vi "Status_Error_Message.vi"(1 "Message number":i32 min=0 step=1) -> (0 "Status/Error string":string)   [LabVIEW 2012]
uses:
  Globals/Status_Error_Messages.vi
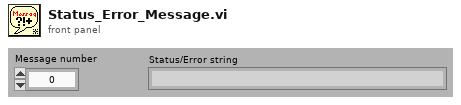
[diagram p1: front panel]
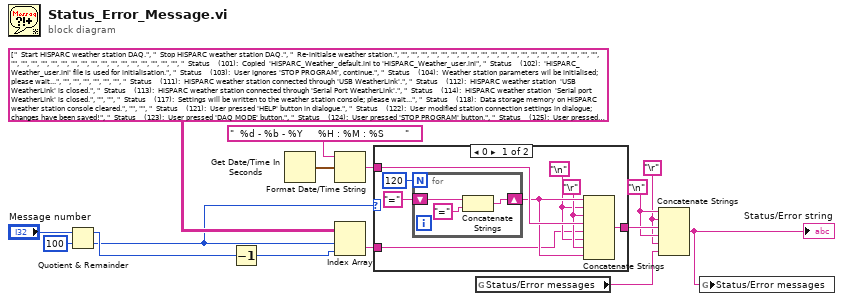
[diagram p0: block diagram]
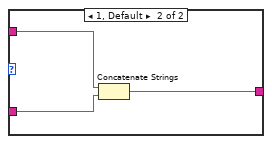
[diagram p2: hidden frame]
diagram:
  w11 = "\n"
  w10 = "\r"
  n1 = Quotient & Remainder(x="Message number", y=100) -> (x-y*floor(x/y)=w5:i32, floor(x/y)=w1:i32)
  n2 = Decrement(x=w5) -> (x-1=w2:i32)
  n3 = Get Date/Time In Seconds() -> (seconds since 1Jan1904=w15:timestamp)
  n4 = Format Date/Time String(time format string (%c)="  %d - %b - %Y     %H : %M : %S       ", seconds (now)=w15) -> (date/time string=w13:string)  [unwired: 1 in]
  n5 = Index Array(array=string[][] [["  Start HiSPARC weather station DAQ.", "  Stop HiSPARC weather station DAQ.", "  Re-initialse weather station.", "", "", "", "", "", "", "", "", "", "", "", "", "", "", "", "", "", "", "", "", "", "", "", "", "", "", "", "", "", "", "", "", "", "", "", "", ""], ["  Status    (101):  Copied  'HiSPARC_Weather_default.ini to 'HiSPARC_Weather_user.ini", "  Status    (102):  'HiSPARC_Weather_user.ini' file is used for initialisation.", "  Status    (103):  User ignores 'STOP PROGRAM', continue.", "  Status    (104):  Weather station parameters wil be initialised; please wait...", "", "", "", "", "", "", "  Status    (111):  HiSPARC weather station connected through 'USB WeatherLink'.", "  Status    (112):  HiSPARC weather station  'USB WeatherLink' is closed.", "  Status    (113):  HiSPARC weather station connected through 'Serial Port WeatherLink'.", "  Status    (114):  HiSPARC weather station  'Serial port WeatherLink' is closed.", "", "", "  Status    (117):  Settings will be written to the weather station console; please wait...", "  Status    (118):  Data storage memory on HiSPARC weather station console cleared.", "", "", "  Status    (121):  User pressed 'HELP' button in dialogue.", "  Status    (122):  User modified station connection settings in dialogue; changes have been saved!", "  Status    (123):  User pressed 'DAQ MODE' button.", "  Status    (124):  User pressed 'STOP PROGRAM' button.", "  Status    (125):  User pressed 'SAVE SETTINGS' button.", "  Status    (126):  User pressed 'SAVE CALIBRATION' button; please wait until settings have been uploaded...", "  Status    (127):  User skips weather station calibration, continue.", "  Status    (128):  User pressed 'RESET' button but skips reset.", "  Status    (129):  User pressed 'HELP' button.", "  Status    (130):  User pressed 'STOP DAQ' button.", "  Status    (131):  Weather station console successfully initialised.", "", "", "", "", "  Status    (136):  Calibration: latitude and longitude have not been modified.", "  Status    (137):  Calibration: temperature and/or humidity settings have not been modified.", "", "  Status    (139):  Calibration: wind direction has not been modified.", "  Status    (140):  Calibration: barometer settings have not been modified."], ["  Warning (201):  No GPS time correction in HiSPARC.ini (correction = 0)!", "", "", "", "", "", "", "", "", "", "  Warning (211):  Cannot open HiSPARC weather station connection through 'USB WeatherLink'!", "  Warning (212):  Cannot close HiSPARC weather station connection through 'USB WeatherLink'", "  Warning (213):  Cannot open HiSPARC weather station connection through 'Serial Port WeatherLink'", "  Warning (214):  Cannot close HiSPARC weather station connection through 'Serial Port WeatherLink'!", "  Warning (215):  Station ID = 0; please choose a valid station number!", "  Warning (216):  Serial COM port number = 0; please choose a valid port number!", "  Warning (217):  Will try to automatically reconnect to HiSPARC weather station!", "  Warning (218):  Could not clear data storage memory on HiSPARC weather station console!", "", "", "  Warning (221):  Please check your internet connection; cannot reach HiSPARC document server!", "  Warning (222):  User pressed 'STOP PROGRAM' button in dialogue!", "  Warning (223):  Overflow event queue for buffer database; 1 event is lost!", "  Warning (224):  Overflow event queue for front panel graphs!", "", "", "  Warning (227):  Latitude, longitude and calibration settings have been transmitted to the console; values stored.", "  Warning (228):  User pressed 'RESET' button; restart with default settings!", "", "  Warning (230):  Failed to initialise weather station console, will retry!", "  Warning (231):  Failed to read weather station DLL/Firmware information and/or clear calibration settings!", "  Warning (232):  Failed to initialise sensor units!", "  Warning (233):  Failed to set rain collector model!", "  Warning (234):  Failed to set wind cup size!", "  Warning (235):  Failed to synchronise pc clock and weather station clock!", "  Warning (236):  Calibration: latitude and/or longitude have been modified.", "  Warning (237):  Calibration: temperature and/or humidity settings have been modified.", "", "  Warning (239):  Calibration: wind direction has been modified.", "  Warning (240):  Calibration: barometer settings have been modified."], ["  Error      (301):  Path to HiSPARC weather station DAQ software has not been found!", "  Error      (302):  Initialisation file 'HiSPARC.ini' has not been found!", "  Error      (303):  Initialisation file 'HiSPARC_Weather_default.ini' has not been found!", "  Error      (304):  Failed copying  'HiSPARC_Weather_default.ini' to 'HiSPARC_Weather_user.ini'!", "  Error      (305):  Path not found to HiSPARC weather station DAQ software!", "  Error      (305):  Error in reading parameters from HiSPARC.ini!", "", "", "", "", "", "", "", "", "", "", "", "", "", "", "", "  Error      (322):  Lost connection to weather station; will automatically try to reconnect!", "  Error      (323):  Cannot connect to database, will automatically return to 'STOP DAQ' mode!", "", "", "", "  Error      (327):  Failed to save 'CALIBRATION' settings.", "", "", "  Error      (330):  Failed to initialise weather station console several times, quit!", "  Error      (331):  The weather station supporting software library (DLL) cannot be initialised!", "  Error      (332):  This weather station model is not supported!", "", "", "", "  Error      (336):  Calibration: failed to set latitude and/or longitude!", "  Error      (337):  Calibration: failed to modify temperature and/or humidity settings!", "  Error      (338):  Calibration: failed to reset temperature and/or humidity calibration settings!", "  Error      (339):  Calibration: failed to modify wind direction!", "  Error      (340):  Calibration: failed to modify barometer settings!"]], index (row)=w1, index (col)=w2) -> (element=w9:string)
  n6 = case shown="0" w1 {
    tunnel: w13 -> [w22 w29]
    tunnel: w9 -> [w17 w28]
    tunnel: [w21 w27] -> w12
    frame 0 {
      w18 = "\n"
      w19 = "\r"
      n7 = for {
        N: 120 -> [_]
        shift-right: [w24] -> w20
        shift-left: "=" -> [w26]
        n8 = Concatenate Strings(w26, "=" ("string")) -> (w24:string)
      }
      n9 = Concatenate Strings(w20, w18, w19, w22, w17, w18, w19, w20) -> (w21:string)
    }
    frame 1, Default {
      n10 = Concatenate Strings(w29, w28) -> (w27:string)
    }
  }
  n11 = global read "Status_Error_Messages.vi" "Status/Error messages"() -> (w4:string)
  n12 = Concatenate Strings(w11, w10, w12, w11, w10, w4) -> (w3:string)
  "Status/Error string" <- w3
  n13 = global write "Status_Error_Messages.vi" "Status/Error messages"(w3) -> ()
